vi "Data Analysis.vi"() -> ()   [LabVIEW 2013]
uses:
  Data Utilities/Analysis Data.ctl
panel:
  in  "nm Between Chains":dbl=28.0
  in  "# Chains":i32=1
  in  "Fit Tabs":enum32{"FJC", "WLC"}(tab)
  in  "Persistence Length (nm)":dbl
  in  "Segment Elasticity (pN/nm)":dbl
  in  "Segment Length (nm)":dbl
  in  "Temperature (K)":dbl=298.0
  in  "Temperature (K)":dbl=298.0
  in  "Persistence Length (nm)":dbl
  out "Slope (nm/V)":dbl format="%#3.3g"
  out "Spring Constant (pN/nm)":dbl format="%#1.1g"
  out "Ramp Rate (nm/s)":dbl format="%#2.2g"
  in  "Save Data":bool
  in  "Clear\nLoaded\nData":bool
  in  "Load Data":bool
  in  "Load Path":path
  in  "Graph Entries":T1
  in  "Adjust Baselines":bool
  out "XY Graph":T2(graph)
  # "Selected Experiment Metadata"
  # "Use square to select, circle to enable."
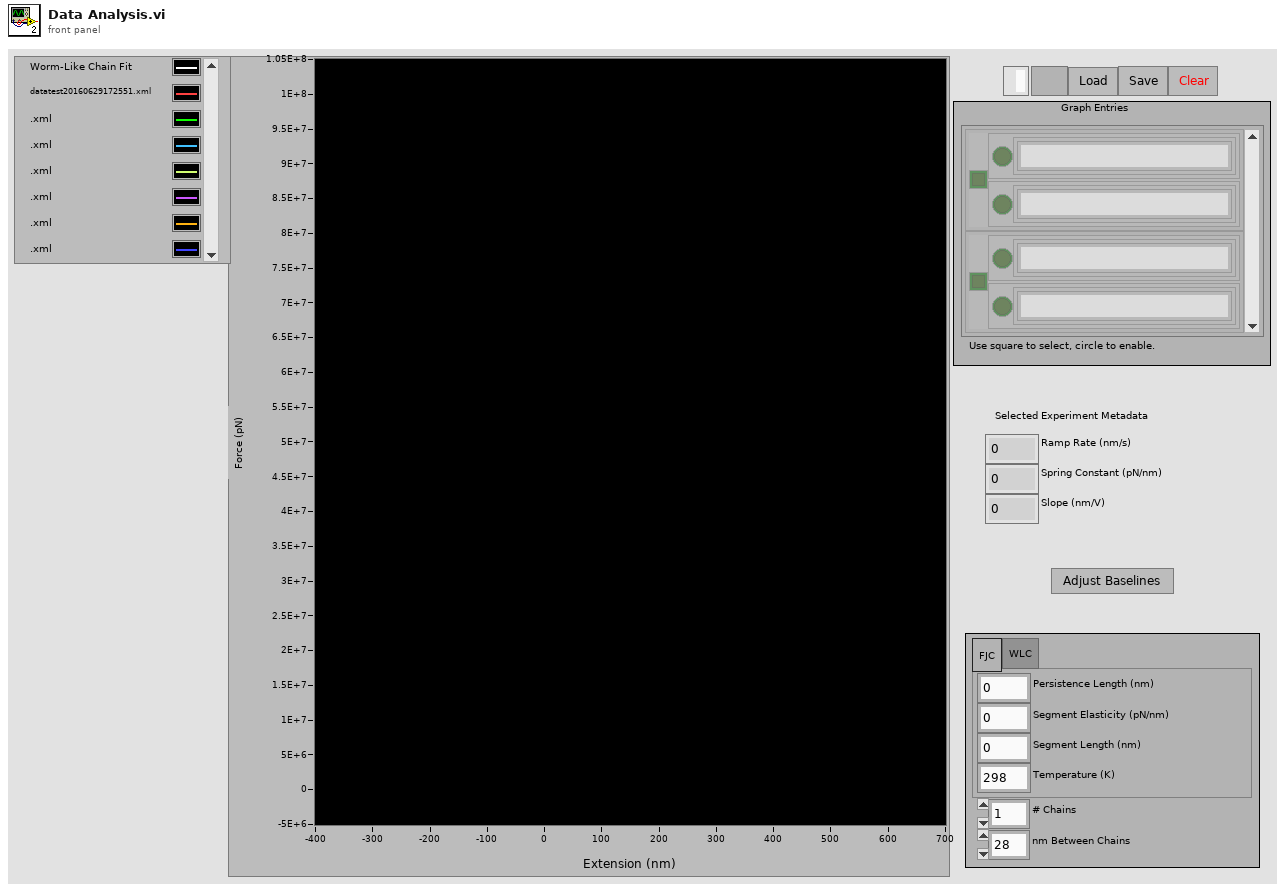
[diagram p1: front panel]
types:
  T1 = typedef "Analysis Data.ctl" = cluster{"Base Directory":path, "Experimental Data":cluster{"Experimental Data":cluster{"Extension (nm)":dbl[], "Force (pN)":dbl[], "Name":string}, "Enabled":bool}, "Chain Fit":cluster{"Experimental Data":cluster{"Extension (nm)":dbl[], "Force (pN)":dbl[], "Name":string}, "Enabled":bool}, "Selected":bool, "Ramp Rate (nm/s)":dbl, "Spring Constant (pN/nm)":dbl, "Slope (nm/V)":dbl}[]
  T2 = cluster{"Extension (nm)":dbl[], "Force (pN)":dbl[]}[]
  T3 = cluster{"Base Directory":path, "Experimental Data":cluster{"Experimental Data":cluster{"Extension (nm)":dbl[], "Force (pN)":dbl[], "Name":string}, "Enabled":bool}, "Chain Fit":cluster{"Experimental Data":cluster{"Extension (nm)":dbl[], "Force (pN)":dbl[], "Name":string}, "Enabled":bool}, "Selected":bool, "Ramp Rate (nm/s)":dbl, "Spring Constant (pN/nm)":dbl, "Slope (nm/V)":dbl}
  T4 = cluster{"Extension (nm)":dbl[], "Force (pN)":dbl[]}
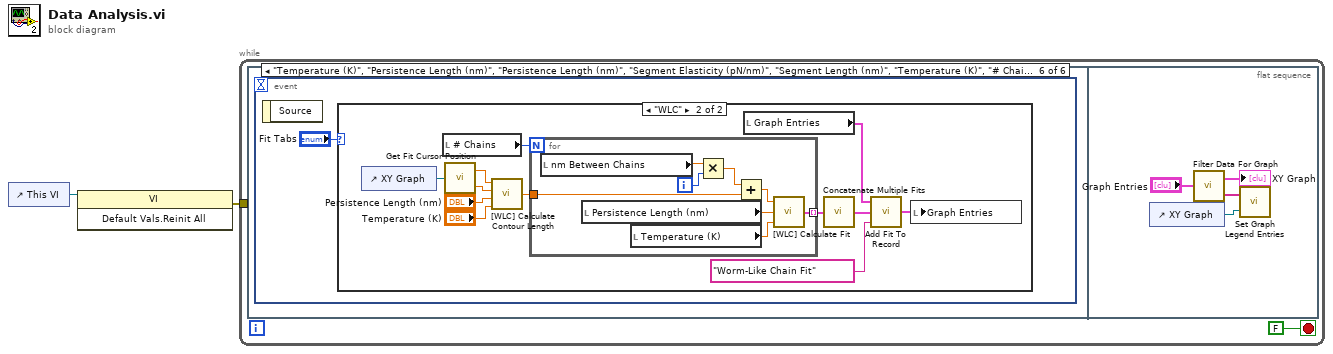
[diagram p0: block diagram]
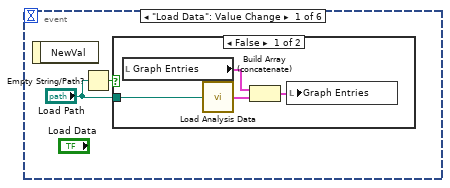
[diagram p2: hidden frame]
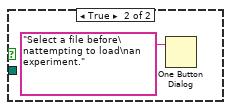
[diagram p3: hidden frame]
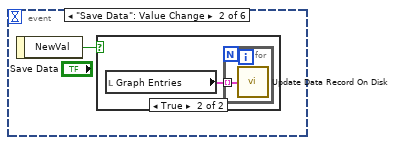
[diagram p4: hidden frame]
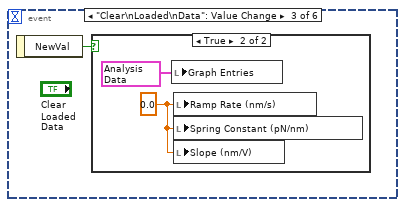
[diagram p6: hidden frame]
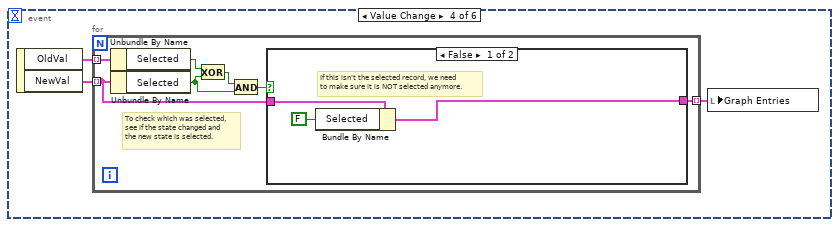
[diagram p8: hidden frame]
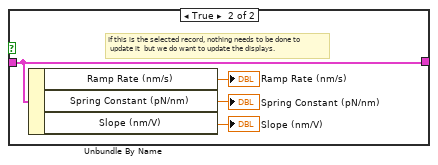
[diagram p9: hidden frame]
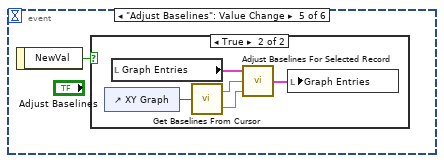
[diagram p10: hidden frame]
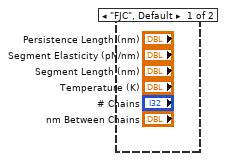
[diagram p12: hidden frame]
diagram:
  n1 = control-ref of="This VI"() -> (w2:refnum<vi>)
  n2 = invoke class="VI" method="Default Vals.Reinit All"(reference=w2) -> (error out=w1:errorcluster)  [unwired: 2 in, 2 out]
  n3 = while {
    tunnel: w1 -> [_]
    stop <- FALSE stop-if-true
    n4 = flat-sequence {
      frame #0 {
        n5 = event shown="[5] \"Temperature (K)\", \"Persistence Length (nm)\", \"Persistence Length (nm)\", \"Segment Elasticity (pN/nm)\", \"Segment Length (nm)\", \"Temperature (K)\", \"# Chains\", \"nm Between Chains\": Value Change" {
          selector: _ -> [_ _ _ _ _ _]
          dyn-events: _ -> [_ _ _ _ _ _]
          timeout: _ -> [_ _ _ _ _ _]
          event "Load Data": Value Change {
            n6 = event-data() -> ()  [unwired: 1 in, 1 out]
            n7 = Empty String/Path?(string/path="Load Path") -> (empty?=w5:bool)
            n8 = case shown="False" w5 {
              tunnel: "Load Path" -> [w7 _]
              frame False {
                n9 = local read "Graph Entries"() -> (w9:T1)
                n10 = call "Load Analysis Data.vi"("Load Path"=w7) -> ("Loaded Entry"=w6:T3)
                n11 = Build Array (concatenate)(w9, w6) -> (w8:T1)
                n12 = local write "Graph Entries"(w8) -> ()
              }
              frame True {
                n13 = One Button Dialog(message="Select a file before\nattempting to load\nan experiment.") -> ()  [unwired: 1 in, 1 out]
              }
            }
          }
          event "Save Data": Value Change {
            n14 = event-data() -> ("NewVal"=w11:bool)  [unwired: 1 in]
            n15 = case shown="True" w11 {
              frame False {
              }
              frame True {
                n16 = local read "Graph Entries"() -> (w12:T1)
                n17 = for {
                  tunnel: w12 -> [w13] mode=indexing
                  n18 = call "Update Data Record On Disk.vi"("Graph Entry"=w13) -> ()
                }
              }
            }
          }
          event "Clear\nLoaded\nData": Value Change {
            n19 = event-data() -> ("NewVal"=w14:bool)  [unwired: 1 in]
            n20 = case shown="True" w14 {
              frame False {
              }
              frame True {
                w15 = 0.0 ("Ramp Rate (nm/s)")
                n21 = local write "Graph Entries"(T1 [{"Base Directory"=path "", "Experimental Data"={"Experimental Data"={"Extension (nm)"=[], "Force (pN)"=[], "Name"=""}, "Enabled"=FALSE}, "Chain Fit"={"Experimental Data"={"Extension (nm)"=[], "Force (pN)"=[], "Name"=""}, "Enabled"=FALSE}, "Selected"=FALSE, "Ramp Rate (nm/s)"=0.0, "Spring Constant (pN/nm)"=0.0, "Slope (nm/V)"=0.0}] ("Graph Entries")) -> ()
                n22 = local write "Ramp Rate (nm/s)"(w15) -> ()
                n23 = local write "Spring Constant (pN/nm)"(w15) -> ()
                n24 = local write "Slope (nm/V)"(w15) -> ()
              }
            }
          }
          event Value Change {
            n25 = event-data() -> ("OldVal"=w19:T1, "NewVal"=w18:T1)  [unwired: 1 in]
            n26 = for {
              tunnel: w19 -> [w26] mode=indexing
              tunnel: w18 -> [w21] mode=indexing
              tunnel: [w20] -> w17 mode=indexing
              # "To check which was selected,\nsee if the state changed and\nthe new state is selected."
              n27 = Unbundle By Name(w26) -> ("Selected"=w24:bool)
              n28 = Unbundle By Name(w21) -> ("Selected"=w23:bool)
              n29 = Exclusive Or(1:w23, 2:w24) -> (0:w25:bool)
              n30 = And(x=w25, y=w23) -> (x .and. y?=w22:bool)
              n31 = case shown="False" w22 {
                tunnel: w21 -> [w29 w33]
                tunnel: [w27 w33] -> w20
                frame False {
                  # "If this isn't the selected record, we need\nto make sure it is NOT selected anymore."
                  n32 = Bundle By Name(cluster=w29, "Selected"=FALSE) -> (w27:T3)
                }
                frame True {
                  # "If this is the selected record, nothing needs to be done to\n update it  but we do want to update the displays."
                  n33 = Unbundle By Name(w33) -> ("Ramp Rate (nm/s)"=→"Ramp Rate (nm/s)":dbl, "Spring Constant (pN/nm)"=→"Spring Constant (pN/nm)":dbl, "Slope (nm/V)"=→"Slope (nm/V)":dbl)
                }
              }
            }
            n34 = local write "Graph Entries"(w17) -> ()
          }
          event "Adjust Baselines": Value Change {
            n35 = event-data() -> ("NewVal"=w34:bool)  [unwired: 1 in]
            n36 = case shown="True" w34 {
              frame False {
              }
              frame True {
                n37 = control-ref of="XY Graph"() -> (w37:refnum<vi>)
                n38 = local read "Graph Entries"() -> (w39:T1)
                n39 = call "Get Baselines From Cursor.vi"("Graph Reference"=w37) -> ("Force Baseline (pN)"=w36:dbl, "Extension Baseline (nm)"=w35:dbl)
                n40 = call "Adjust Baselines For Selected Record.vi"("Extension Baseline (nm)"=w35, "Force Baseline (pN)"=w36, "Input State"=w39) -> ("Adjusted State"=w38:T1)
                n41 = local write "Graph Entries"(w38) -> ()
              }
            }
          }
          event "Temperature (K)", "Persistence Length (nm)", "Persistence Length (nm)", "Segment Elasticity (pN/nm)", "Segment Length (nm)", "Temperature (K)", "# Chains", "nm Between Chains": Value Change {
            n42 = event-data() -> ()  [unwired: 1 in, 1 out]
            n43 = case shown="\"WLC\"" "Fit Tabs" {
              frame "FJC", Default {
              }
              frame "WLC" {
                n44 = control-ref of="XY Graph"() -> (w42:refnum<vi>)
                n45 = local read "# Chains"() -> (w48:i32)
                n46 = call "Get Fit Cursor Position.vi"("Graph Reference"=w42) -> ("Force (pN)"=w50:dbl, "Extension (nm)"=w52:dbl)
                n47 = call "[WLC] Calculate Contour Length.vi"("Temperature (K)"="Temperature (K)", "Persistence Length (nm)"="Persistence Length (nm)", "Extension (nm)"=w52, "Force (pN)"=w50) -> ("Contour Length (nm)"=w47:dbl)
                n48 = for {
                  N: w48 -> [_]
                  tunnel: w47 -> [w58]
                  tunnel: [w53] -> w46 mode=indexing
                  i -> [w60]
                  n49 = local read "nm Between Chains"() -> (w59:dbl)
                  n50 = local read "Persistence Length (nm)"() -> (w56:dbl)
                  n51 = local read "Temperature (K)"() -> (w54:dbl)
                  n52 = Multiply(x=w59, y=w60) -> (x*y=w57:dbl)
                  n53 = Add(x=w57, y=w58) -> (x+y=w55:dbl)
                  n54 = call "[WLC] Calculate Fit.vi"("Temperature (K)"=w54, "Persistence Length (nm)"=w56, "Contour Length (nm)"=w55) -> ("Worm-Like Chain Fit"=w53:T4)
                }
                n55 = local read "Graph Entries"() -> (w43:T1)
                n56 = call "Concatenate Multiple Fits.vi"("Fits"=w46) -> ("Concatenated Fits"=w45:cluster{dbl[], dbl[]})
                n57 = call "Add Fit To Record.vi"("Fit Name"="Worm-Like Chain Fit", "Chain Fit"=w45, "Input State"=w43) -> ("State With Fit"=w41:T1)
                n58 = local write "Graph Entries"(w41) -> ()
              }
            }
          }
        }
      }
      frame #1 {
        n59 = control-ref of="XY Graph"() -> (w61:refnum<vi>)
        n60 = call "Filter Data For Graph.vi"("Input State"="Graph Entries") -> ("Graph Entries"=→"XY Graph":T2, "Legend Entries"=w62:string[])
        n61 = call "Set Graph Legend Entries.vi"("Graph Reference"=w61, "Legend Entries"=w62) -> ()
      }
    }
  }
